vi "Panel Size change (SubVI).vi"(7 "Value":bool, 9 "Bottom":i16, 10 "Right":i16, 11 "Boolean in":refnum<vi>) -> (2 "Numeric 2":i16, 3 "Numeric":i16)   [LabVIEW 2013]
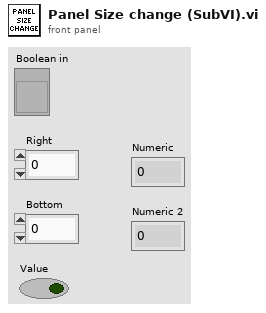
[diagram p1: front panel]
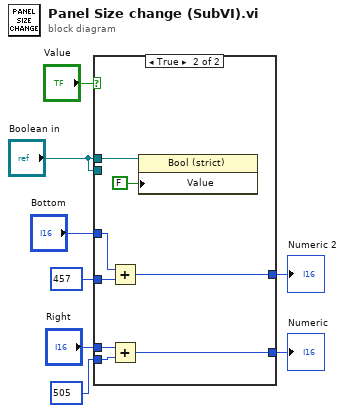
[diagram p0: block diagram]
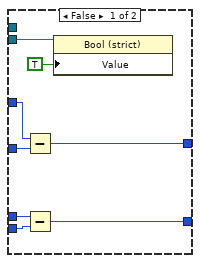
[diagram p2: hidden frame]
diagram:
  n1 = case shown="True" "Value" {
    tunnel: "Bottom" -> [w16 w24]
    tunnel: [w15 w23] -> w3
    tunnel: [w13 w21] -> w5
    tunnel: "Right" -> [w14 w20]
    tunnel: i16 457 ("y 3") -> [w11 w18]
    tunnel: i16 505 ("y 3") -> [w10 w19]
    tunnel: "Boolean in" -> [w9 _]
    tunnel: "Boolean in" -> [_ w17]
    frame False {
      n2 = Subtract(x=w16, y=w11) -> (x-y=w15:i16)
      n3 = Subtract(x=w14, y=w10) -> (x-y=w13:i16)
      n4 = property on="Property Node" class="Bool (strict)"(reference=w9, "Value"=TRUE ("resize Fl")) -> ()  [unwired: 1 in, 2 out]
    }
    frame True {
      n5 = Add(x=w24, y=w18) -> (x+y=w23:i16)
      n6 = Add(x=w20, y=w19) -> (x+y=w21:i16)
      n7 = property on="Property Node" class="Bool (strict)"(reference=w17, "Value"=FALSE ("resize Fl")) -> ()  [unwired: 1 in, 2 out]
    }
  }
  "Numeric" <- w5
  "Numeric 2" <- w3
